vi "Read All Status.vi"(8 "error in (no error)":errorcluster, 10 "Lamps In":T1, 11 "Lamp Container in":refnum<class "Lamp Container.lvclass">) -> (0 "error out":errorcluster, 2 "Lamps Out":T1, 3 "Lamp Container out":refnum<class "Lamp Container.lvclass">)   [LabVIEW 2016, in "Lamp Container.lvclass"]
uses:
  Lamp Container.lvclass
  Controls/Lamps.ctl
  Lamp Container.lvclass/Lamp Container.ctl
  ThAr/ThAr.lvclass
  LED/LED.lvclass
  Quartz/Quartz.lvclass
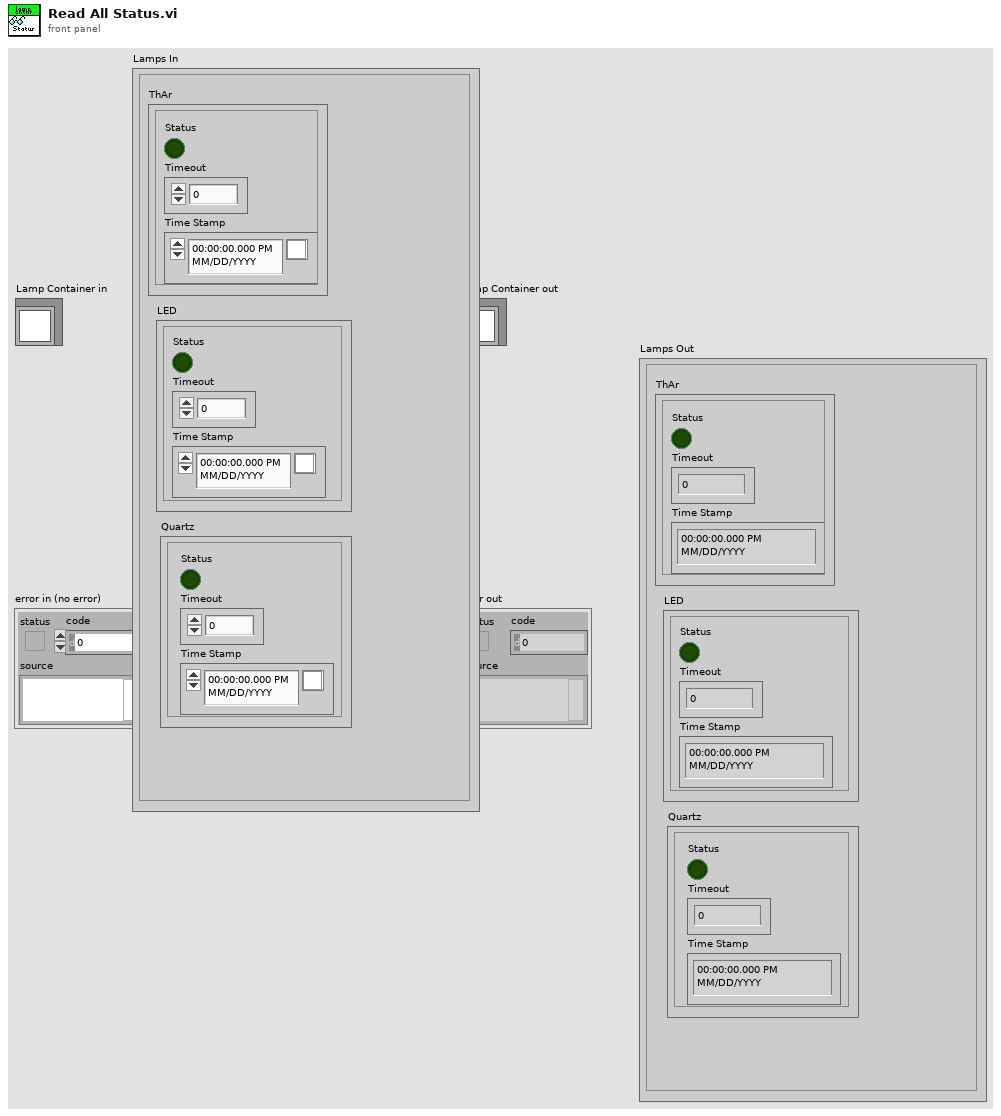
[diagram p1: front panel]
types:
  T1 = typedef "Lamps.ctl" = cluster{"ThAr":cluster{"Time Stamp":timestamp, "Status":bool, "Timeout":dbl}, "LED":cluster{"Time Stamp":timestamp, "Status":bool, "Timeout":dbl}, "Quartz":cluster{"Time Stamp":timestamp, "Status":bool, "Timeout":dbl}}
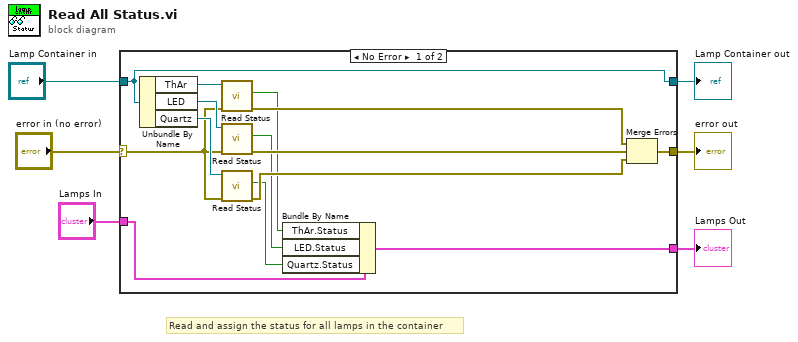
[diagram p0: block diagram]
diagram:
  # "Read and assign the status for all lamps in the container"
  n1 = case shown="No Error" "error in (no error)" {
    selector: "error in (no error)" -> [w7 w23]
    tunnel: [w17 w23] -> w5
    tunnel: [w9 w22] -> w3
    tunnel: "Lamp Container in" -> [w9 w22]
    tunnel: "Lamps In" -> [w13 w21]
    tunnel: [w8 w21] -> w1
    frame No Error {
      n2 = Unbundle By Name(w9) -> ("ThAr"=w20:refnum<class "ThAr.lvclass">, "LED"=w19:refnum<class "LED.lvclass">, "Quartz"=w18:refnum<class "Quartz.lvclass">)
      n3 = call-dynamic "Read Status.vi"("error in (no error)"=w7, "Lamp in"=w20) -> ("error out"=w14:errorcluster, "Status"=w12:bool)  [unwired: 7 in, 1 out]
      n4 = call-dynamic "Read Status.vi"("error in (no error)"=w7, "Lamp in"=w19) -> ("error out"=w15:errorcluster, "Status"=w11:bool)  [unwired: 7 in, 1 out]
      n5 = call-dynamic "Read Status.vi"("error in (no error)"=w7, "Lamp in"=w18) -> ("error out"=w16:errorcluster, "Status"=w10:bool)  [unwired: 7 in, 1 out]
      n6 = Bundle By Name(cluster=w13, "ThAr.Status"=w12, "LED.Status"=w11, "Quartz.Status"=w10) -> (w8:T1)
      n7 = Merge Errors(w14, w15, w16) -> (w17:errorcluster)
    }
    frame Error {
    }
  }
  "error out" <- w5
  "Lamp Container out" <- w3
  "Lamps Out" <- w1
